vi "PicoScope4000aGetRapidBlockBulk.vi"(0 "error in":errorcluster, 3 "handle in":i16, 4 "Enabled array":i16[](array[numeric]), 5 "Rapid Block Acquisition Settings":T1) -> (6 "Channel A Buffer":i16[][](array[numeric]), 7 "Channel E Buffer":i16[][](array[numeric]), 8 "Channel B Buffer":i16[][](array[numeric]), 9 "Channel F Buffer":i16[][](array[numeric]), 10 "Channel C Buffer":i16[][](array[numeric]), 11 "Channel G Buffer":i16[][](array[numeric]), 12 "Channel D Buffer":i16[][](array[numeric]), 13 "Channel H Buffer":i16[][](array[numeric]), 14 "error out":errorcluster, 15 "handle out":i16, 16 "overflow":i16[](array[numeric]) format="%08b", 19 "Num samples":u32)   [LabVIEW 2009]
doc: "This VI gets a set of blocks captured using rapid block mode. It outputs two-dimensional arrays for each channel that contain data from all the requested captures."
uses:
  ps4000a.dll
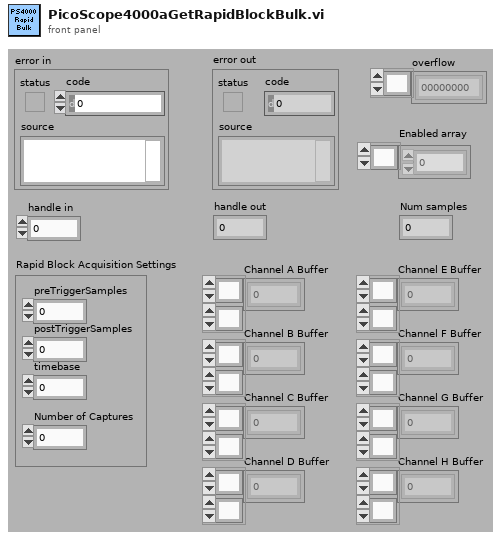
[diagram p1: front panel]
types:
  T1 = cluster{"preTriggerSamples":i32, "postTriggerSamples":i32, "timebase":u32, "Number of Captures":u32}
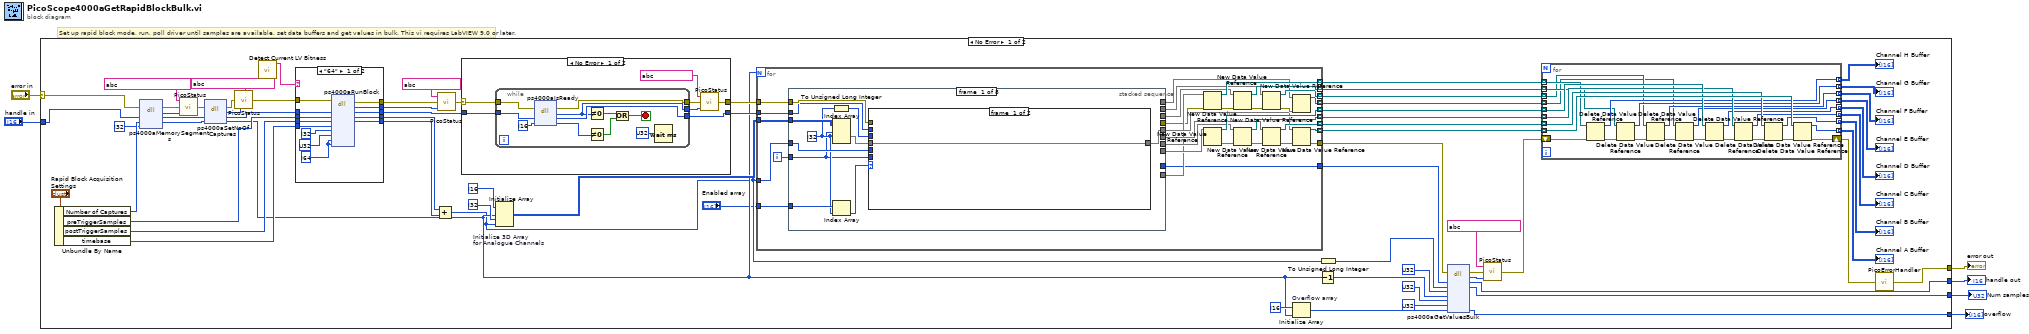
[diagram p0: block diagram]
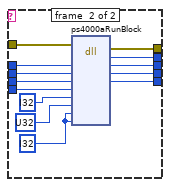
[diagram p2: hidden frame]
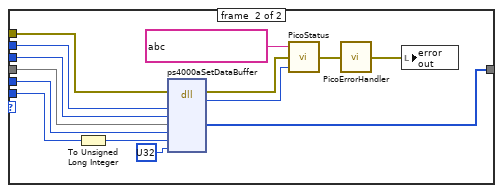
[diagram p3: hidden frame]
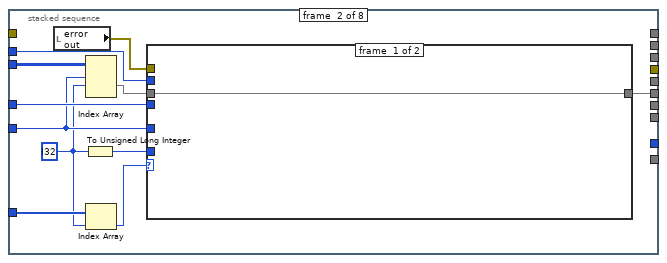
[diagram p4: hidden frame]
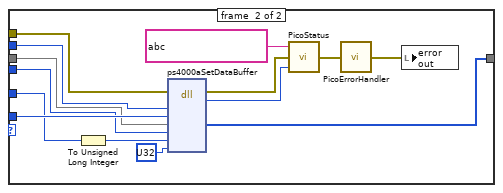
[diagram p5: hidden frame]
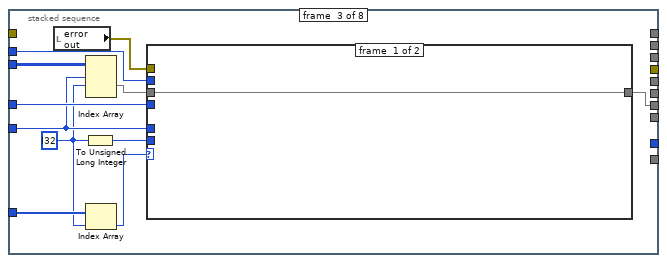
[diagram p6: hidden frame]
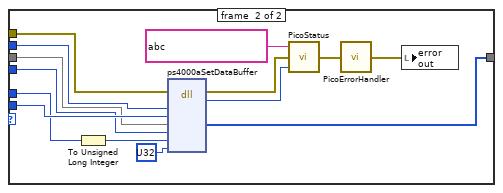
[diagram p7: hidden frame]
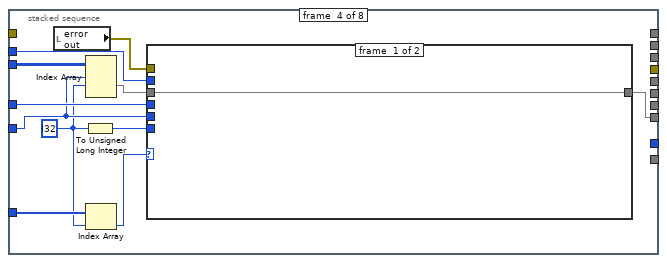
[diagram p8: hidden frame]
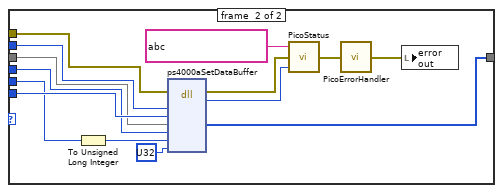
[diagram p9: hidden frame]
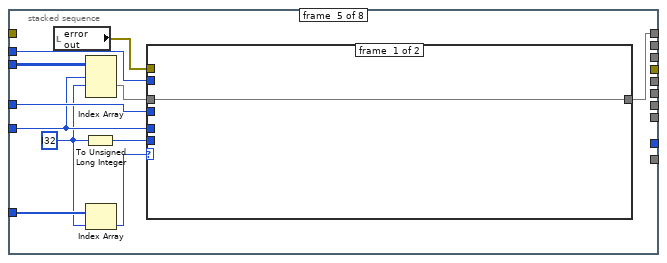
[diagram p10: hidden frame]
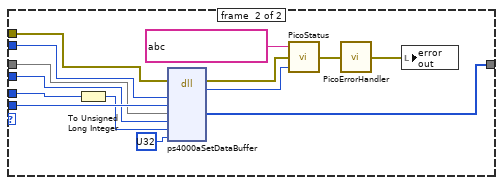
[diagram p11: hidden frame]
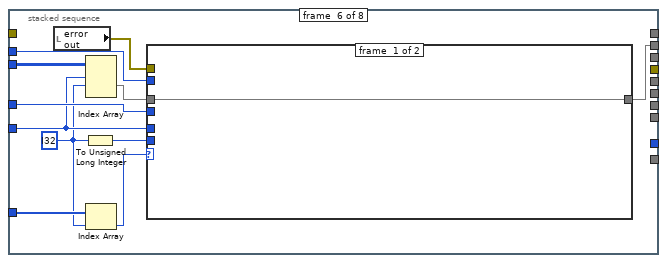
[diagram p12: hidden frame]
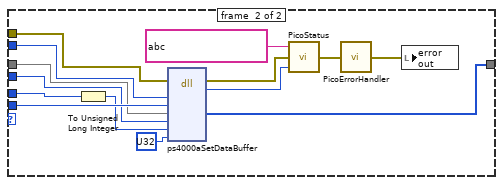
[diagram p13: hidden frame]
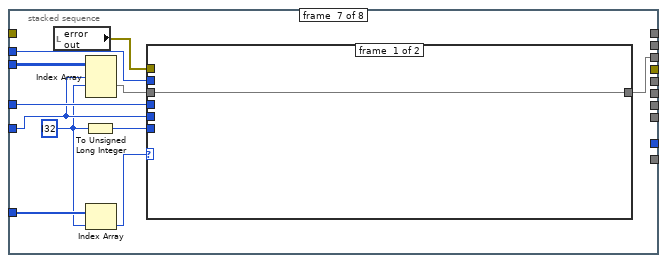
[diagram p14: hidden frame]
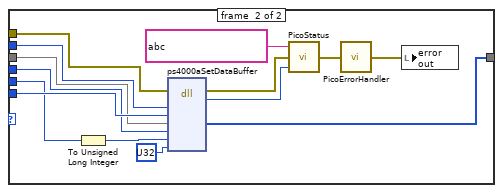
[diagram p15: hidden frame]
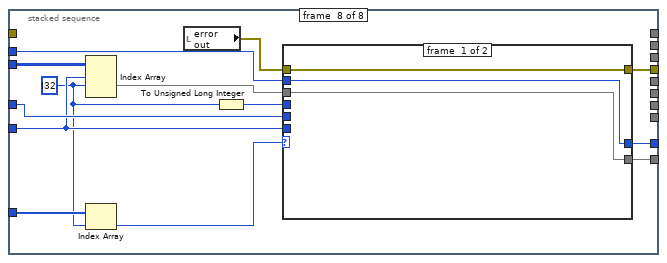
[diagram p16: hidden frame]
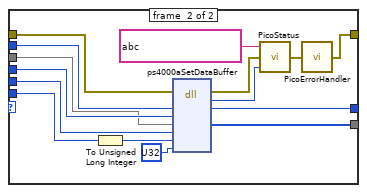
[diagram p17: hidden frame]
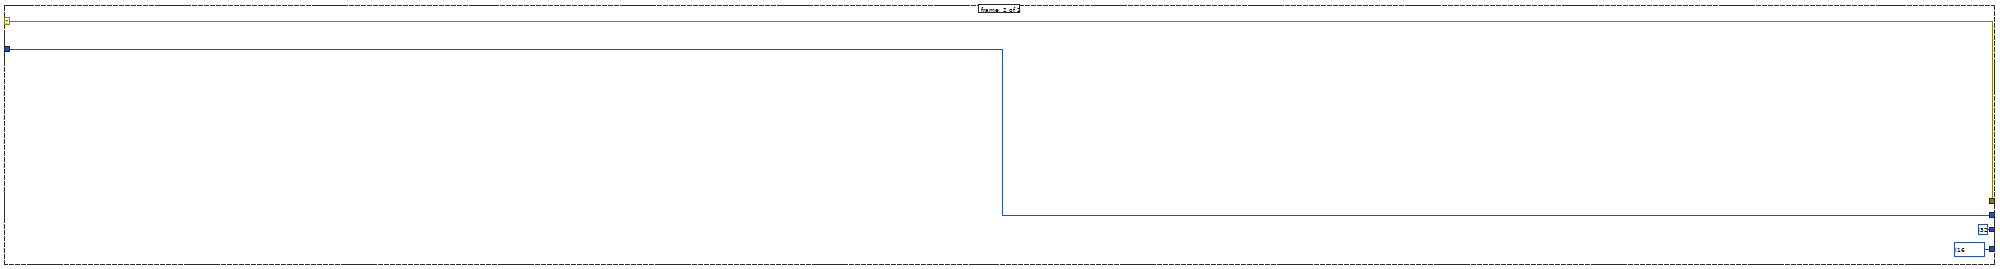
[diagram p19: hidden frame]
diagram:
  # "Set up rapid block mode, run, poll driver until samples are available, set data buffers and get values in bulk. This vi requires LabVIEW 9.0 or later."
  n1 = case shown="No Error" "error in" {
    selector: "error in" -> [w62 w394]
    tunnel: [w47 w394] -> w5
    tunnel: "handle in" -> [w61 w393]
    tunnel: [w37 w393] -> w3
    tunnel: [w19 i32 ?] -> w2
    tunnel: [w8 i16[] ? ("overflow")] -> w1
    frame #0 {
      n2 = Unbundle By Name("Rapid Block Acquisition Settings") -> ("Number of Captures"=w57:u32, "preTriggerSamples"=w68:i32, "postTriggerSamples"=w67:i32, "timebase"=w69:u32)
      n3 = dll-call lib="ps4000a.dll" fn="ps4000aMemorySegments" ("ps3000.dll:_ps3000_open_unit@0")(error in=w62, "handle"=w61, "nSegments"=w57, "nMaxSamples"=i32 ?) -> (error out=w59:errorcluster, "PICO_STATUS"=w60:u32, "handle"=w54:i16, "nSegments"=w55:u32)  [unwired: 3 in, 1 out]
      n4 = call "PicoStatus.vi"("PICO STATUS"=w60, "error in"=w59, "source"=string ?) -> ("error out"=w53:errorcluster)
      n5 = dll-call lib="ps4000a.dll" fn="ps4000aSetNoOfCaptures" ("ps3000.dll:_ps3000_open_unit@0")(error in=w53, "handle"=w54, "nCaptures"=w55) -> (error out=w51:errorcluster, "PICO_STATUS"=w52:u32, "handle"=w48:i16, "nCaptures"=w21:u32)  [unwired: 2 in, 1 out]
      n6 = call "PicoStatus.vi"("PICO STATUS"=w52, "error in"=w51, "source"=string ?) -> ("error out"=w49:errorcluster)
      n7 = call "Detect Current LV Bitness.vi"() -> ("bitness"=w7:string)  [unwired: 11 in]
      n8 = case shown="\"64\"" w7 {
        tunnel: [w88 w101] -> w75
        tunnel: [w87 w100] -> w73
        tunnel: [w86 w99] -> w72
        tunnel: w69 -> [w85 w98]
        tunnel: w68 -> [w84 w97]
        tunnel: w67 -> [w83 w96]
        tunnel: [w82 w95] -> w66
        tunnel: [w81 w94] -> w65
        tunnel: w49 -> [w80 w93]
        tunnel: w48 -> [w79 w92]
        frame #0 {
          w76 = i64 ? ("pParameter")
          n9 = dll-call lib="ps4000a.dll" fn="ps4000aRunBlock" ("ps3000.dll:_ps3000_open_unit@0")(error in=w80, "handle"=w79, "preTriggerSamples"=w84, "postTriggerSamples"=w83, "timebase"=w85, "timeindisposedMs"=i32 ? ("pParameter"), "segmentIndex"=u32 ? ("pParameter"), "lpReady"=w76, "pParameter"=w76) -> (error out=w81:errorcluster, "PICO_STATUS"=w82:u32, "handle"=w88:i16, "preTriggerSamples"=w87:i32, "postTriggerSamples"=w86:i32)  [unwired: 7 in, 1 out]
        }
        frame #1 {
          w89 = i32 ? ("pParameter")
          n10 = dll-call lib="ps4000a.dll" fn="ps4000aRunBlock" ("ps3000.dll:_ps3000_open_unit@0")(error in=w93, "handle"=w92, "preTriggerSamples"=w97, "postTriggerSamples"=w96, "timebase"=w98, "timeindisposedMs"=i32 ? ("pParameter"), "segmentIndex"=u32 ? ("pParameter"), "lpReady"=w89, "pParameter"=w89) -> (error out=w94:errorcluster, "PICO_STATUS"=w95:u32, "handle"=w101:i16, "preTriggerSamples"=w100:i32, "postTriggerSamples"=w99:i32)  [unwired: 7 in, 1 out]
        }
      }
      n11 = Add(x=w73, y=w72) -> (x+y=w20:i32)
      n12 = call "PicoStatus.vi"("PICO STATUS"=w66, "error in"=w65, "source"=string ?) -> ("error out"=w64:errorcluster)
      n13 = case shown="No Error" w64 {
        selector: w64 -> [w375 w389]
        tunnel: w75 -> [w377 w390]
        tunnel: [w376 w390] -> w74
        tunnel: [w374 w389] -> w71
        frame #0 {
          n14 = while {
            tunnel: [w388] -> w376
            tunnel: w377 -> [w387]
            tunnel: [w382] -> w372
            tunnel: w375 -> [w381]
            tunnel: [w380] -> w373
            stop <- w386 stop-if-true
            n15 = dll-call lib="ps4000a.dll" fn="ps4000aIsReady" ("ps3000.dll:_ps3000_open_unit@0")(error in=w381, "handle"=w387, "ready"=i16 ?) -> (error out=w380:errorcluster, "PICO_STATUS"=w382:u32, "handle"=w388:i16, "ready"=w383:i16)  [unwired: 2 in, 1 out]
            n16 = Not Equal To 0?(x=w382) -> (x != 0?=w384:bool)
            n17 = Not Equal To 0?(x=w383) -> (x != 0?=w385:bool)
            n18 = Or(x=w384, y=w385) -> (x .or. y?=w386:bool)
            n19 = Wait (ms)(milliseconds to wait=u32 ? ("ready")) -> ()  [unwired: 1 out]
          }
          n20 = call "PicoStatus.vi"("PICO STATUS"=w372, "error in"=w373, "source"=string ?) -> ("error out"=w374:errorcluster)
        }
        frame #1 {
        }
      }
      n21 = Initialize Array "Initialize 3D Array\nfor Analogue Channels"(i16 ? ("element"), w21, i32 ? ("dimension size"), w20) -> (w22:i16[][][])
      n22 = for {
        N: w21 -> [_]
        tunnel: w74 -> [w137]
        tunnel: w71 -> [w141]
        tunnel: [w150] -> w36
        tunnel: [w154] -> w35 mode=indexing
        tunnel: [w153] -> w34 mode=indexing
        tunnel: [w152] -> w33 mode=indexing
        tunnel: [w151] -> w32 mode=indexing
        tunnel: [w127] -> w28
        tunnel: w22 -> [w139]
        tunnel: w20 -> [w138]
        tunnel: [w146] -> w13 mode=indexing
        tunnel: [w145] -> w12 mode=indexing
        tunnel: [w144] -> w11 mode=indexing
        tunnel: [w143] -> w10 mode=indexing
        tunnel: "Enabled array" -> [w142]
        i -> [w140]
        n23 = stacked-sequence {
          tunnel: [w166 _ _ _ _ _ _ _] -> w136
          tunnel: w142 -> [w168 w194 w220 w246 w272 w298 w324 w352]
          tunnel: w141 -> [w164 _ _ _ _ _ _ _]
          tunnel: w140 -> [w158 w186 w212 w238 w264 w290 w316 w344]
          tunnel: w139 -> [w163 w191 w217 w243 w269 w295 w321 w349]
          tunnel: w138 -> [w161 w189 w215 w241 w267 w293 w319 w347]
          tunnel: w137 -> [w160 w188 w214 w240 w266 w292 w318 w346]
          tunnel: [_ w184 _ _ _ _ _ _] -> w135
          tunnel: [_ _ w210 _ _ _ _ _] -> w134
          tunnel: [_ _ _ w236 _ _ _ _] -> w133
          tunnel: [_ _ _ _ w262 _ _ _] -> w132
          tunnel: [_ _ _ _ _ w288 _ _] -> w131
          tunnel: [_ _ _ _ _ _ w314 _] -> w130
          tunnel: [_ _ _ _ _ _ _ w342] -> w129
          tunnel: [_ _ _ _ _ _ _ w341] -> w128
          tunnel: [_ _ _ _ _ _ _ w340] -> w127
          frame #0 {
            w159 = i32 ? ("index")
            n24 = To Unsigned Long Integer(number=w159) -> (unsigned 32bit integer=w165:u32)
            n25 = Index Array(array=w163, index (dim 0)=w158, index (dim 1)=w159) -> (element=w162:i16[])  [unwired: 1 in]
            n26 = Index Array(array=w168, index=w159) -> (element=w167:i16)
            n27 = case shown="1" w167 {
              tunnel: w164 -> [_ w180]
              tunnel: [w169 w179] -> w166
              tunnel: w165 -> [_ w176]
              tunnel: w162 -> [w169 w174]
              tunnel: w161 -> [_ w173]
              tunnel: w158 -> [_ w172]
              tunnel: w160 -> [_ w170]
              frame #0 {
              }
              frame #1 {
                n28 = To Unsigned Long Integer(number=w172) -> (unsigned 32bit integer=w171:u32)
                n29 = dll-call lib="ps4000a.dll" fn="ps4000aSetDataBuffer" ("ps3000.dll:_ps3000_open_unit@0")(error in=w180, "handle"=w170, "channel"=w176, "buffer"=w174, "bufferLth"=w173, "segmentIndex"=w171, "mode"=u32 ?) -> (error out=w183:errorcluster, "PICO_STATUS"=w182:u32, "buffer"=w179:i16[])  [unwired: 7 in, 1 out]
                n30 = call "PicoStatus.vi"("PICO STATUS"=w182, "error in"=w183, "source"=string ?) -> ("error out"=w178:errorcluster)
                n31 = call "PicoErrorHandler.vi"("error in"=w178) -> ("error out"=w175:errorcluster)
                n32 = local write "error out"(w175) -> ()
              }
            }
          }
          frame #1 {
            w185 = i32 ? ("index")
            n33 = local read "error out"() -> (w187:errorcluster)
            n34 = To Unsigned Long Integer(number=w185) -> (unsigned 32bit integer=w192:u32)
            n35 = Index Array(array=w191, index (dim 0)=w186, index (dim 1)=w185) -> (element=w190:i16[])  [unwired: 1 in]
            n36 = Index Array(array=w194, index=w185) -> (element=w193:i16)
            n37 = case shown="1" w193 {
              tunnel: w187 -> [_ w206]
              tunnel: [w195 w205] -> w184
              tunnel: w192 -> [_ w202]
              tunnel: w190 -> [w195 w200]
              tunnel: w189 -> [_ w199]
              tunnel: w186 -> [_ w198]
              tunnel: w188 -> [_ w196]
              frame #0 {
              }
              frame #1 {
                n38 = To Unsigned Long Integer(number=w198) -> (unsigned 32bit integer=w197:u32)
                n39 = dll-call lib="ps4000a.dll" fn="ps4000aSetDataBuffer" ("ps3000.dll:_ps3000_open_unit@0")(error in=w206, "handle"=w196, "channel"=w202, "buffer"=w200, "bufferLth"=w199, "segmentIndex"=w197, "mode"=u32 ?) -> (error out=w209:errorcluster, "PICO_STATUS"=w208:u32, "buffer"=w205:i16[])  [unwired: 7 in, 1 out]
                n40 = call "PicoStatus.vi"("PICO STATUS"=w208, "error in"=w209, "source"=string ?) -> ("error out"=w204:errorcluster)
                n41 = call "PicoErrorHandler.vi"("error in"=w204) -> ("error out"=w201:errorcluster)
                n42 = local write "error out"(w201) -> ()
              }
            }
          }
          frame #2 {
            w211 = i32 ? ("index")
            n43 = local read "error out"() -> (w213:errorcluster)
            n44 = To Unsigned Long Integer(number=w211) -> (unsigned 32bit integer=w218:u32)
            n45 = Index Array(array=w217, index (dim 0)=w212, index (dim 1)=w211) -> (element=w216:i16[])  [unwired: 1 in]
            n46 = Index Array(array=w220, index=w211) -> (element=w219:i16)
            n47 = case shown="1" w219 {
              tunnel: w213 -> [_ w232]
              tunnel: [w221 w231] -> w210
              tunnel: w218 -> [_ w228]
              tunnel: w216 -> [w221 w226]
              tunnel: w215 -> [_ w225]
              tunnel: w212 -> [_ w224]
              tunnel: w214 -> [_ w222]
              frame #0 {
              }
              frame #1 {
                n48 = To Unsigned Long Integer(number=w224) -> (unsigned 32bit integer=w223:u32)
                n49 = dll-call lib="ps4000a.dll" fn="ps4000aSetDataBuffer" ("ps3000.dll:_ps3000_open_unit@0")(error in=w232, "handle"=w222, "channel"=w228, "buffer"=w226, "bufferLth"=w225, "segmentIndex"=w223, "mode"=u32 ?) -> (error out=w235:errorcluster, "PICO_STATUS"=w234:u32, "buffer"=w231:i16[])  [unwired: 7 in, 1 out]
                n50 = call "PicoStatus.vi"("PICO STATUS"=w234, "error in"=w235, "source"=string ?) -> ("error out"=w230:errorcluster)
                n51 = call "PicoErrorHandler.vi"("error in"=w230) -> ("error out"=w227:errorcluster)
                n52 = local write "error out"(w227) -> ()
              }
            }
          }
          frame #3 {
            w237 = i32 ? ("index")
            n53 = local read "error out"() -> (w239:errorcluster)
            n54 = To Unsigned Long Integer(number=w237) -> (unsigned 32bit integer=w244:u32)
            n55 = Index Array(array=w243, index (dim 0)=w238, index (dim 1)=w237) -> (element=w242:i16[])  [unwired: 1 in]
            n56 = Index Array(array=w246, index=w237) -> (element=w245:i16)
            n57 = case shown="1" w245 {
              tunnel: w239 -> [_ w258]
              tunnel: [w247 w257] -> w236
              tunnel: w244 -> [_ w254]
              tunnel: w242 -> [w247 w252]
              tunnel: w241 -> [_ w251]
              tunnel: w238 -> [_ w250]
              tunnel: w240 -> [_ w248]
              frame #0 {
              }
              frame #1 {
                n58 = To Unsigned Long Integer(number=w250) -> (unsigned 32bit integer=w249:u32)
                n59 = dll-call lib="ps4000a.dll" fn="ps4000aSetDataBuffer" ("ps3000.dll:_ps3000_open_unit@0")(error in=w258, "handle"=w248, "channel"=w254, "buffer"=w252, "bufferLth"=w251, "segmentIndex"=w249, "mode"=u32 ?) -> (error out=w261:errorcluster, "PICO_STATUS"=w260:u32, "buffer"=w257:i16[])  [unwired: 7 in, 1 out]
                n60 = call "PicoStatus.vi"("PICO STATUS"=w260, "error in"=w261, "source"=string ?) -> ("error out"=w256:errorcluster)
                n61 = call "PicoErrorHandler.vi"("error in"=w256) -> ("error out"=w253:errorcluster)
                n62 = local write "error out"(w253) -> ()
              }
            }
          }
          frame #4 {
            w263 = i32 ? ("index")
            n63 = local read "error out"() -> (w265:errorcluster)
            n64 = To Unsigned Long Integer(number=w263) -> (unsigned 32bit integer=w270:u32)
            n65 = Index Array(array=w269, index (dim 0)=w264, index (dim 1)=w263) -> (element=w268:i16[])  [unwired: 1 in]
            n66 = Index Array(array=w272, index=w263) -> (element=w271:i16)
            n67 = case shown="1" w271 {
              tunnel: w265 -> [_ w284]
              tunnel: [w273 w283] -> w262
              tunnel: w270 -> [_ w280]
              tunnel: w268 -> [w273 w278]
              tunnel: w267 -> [_ w277]
              tunnel: w264 -> [_ w276]
              tunnel: w266 -> [_ w274]
              frame #0 {
              }
              frame #1 {
                n68 = To Unsigned Long Integer(number=w276) -> (unsigned 32bit integer=w275:u32)
                n69 = dll-call lib="ps4000a.dll" fn="ps4000aSetDataBuffer" ("ps3000.dll:_ps3000_open_unit@0")(error in=w284, "handle"=w274, "channel"=w280, "buffer"=w278, "bufferLth"=w277, "segmentIndex"=w275, "mode"=u32 ?) -> (error out=w287:errorcluster, "PICO_STATUS"=w286:u32, "buffer"=w283:i16[])  [unwired: 7 in, 1 out]
                n70 = call "PicoStatus.vi"("PICO STATUS"=w286, "error in"=w287, "source"=string ?) -> ("error out"=w282:errorcluster)
                n71 = call "PicoErrorHandler.vi"("error in"=w282) -> ("error out"=w279:errorcluster)
                n72 = local write "error out"(w279) -> ()
              }
            }
          }
          frame #5 {
            w289 = i32 ? ("index")
            n73 = local read "error out"() -> (w291:errorcluster)
            n74 = To Unsigned Long Integer(number=w289) -> (unsigned 32bit integer=w296:u32)
            n75 = Index Array(array=w295, index (dim 0)=w290, index (dim 1)=w289) -> (element=w294:i16[])  [unwired: 1 in]
            n76 = Index Array(array=w298, index=w289) -> (element=w297:i16)
            n77 = case shown="1" w297 {
              tunnel: w291 -> [_ w310]
              tunnel: [w299 w309] -> w288
              tunnel: w296 -> [_ w306]
              tunnel: w294 -> [w299 w304]
              tunnel: w293 -> [_ w303]
              tunnel: w290 -> [_ w302]
              tunnel: w292 -> [_ w300]
              frame #0 {
              }
              frame #1 {
                n78 = To Unsigned Long Integer(number=w302) -> (unsigned 32bit integer=w301:u32)
                n79 = dll-call lib="ps4000a.dll" fn="ps4000aSetDataBuffer" ("ps3000.dll:_ps3000_open_unit@0")(error in=w310, "handle"=w300, "channel"=w306, "buffer"=w304, "bufferLth"=w303, "segmentIndex"=w301, "mode"=u32 ?) -> (error out=w313:errorcluster, "PICO_STATUS"=w312:u32, "buffer"=w309:i16[])  [unwired: 7 in, 1 out]
                n80 = call "PicoStatus.vi"("PICO STATUS"=w312, "error in"=w313, "source"=string ?) -> ("error out"=w308:errorcluster)
                n81 = call "PicoErrorHandler.vi"("error in"=w308) -> ("error out"=w305:errorcluster)
                n82 = local write "error out"(w305) -> ()
              }
            }
          }
          frame #6 {
            w315 = i32 ? ("index")
            n83 = local read "error out"() -> (w317:errorcluster)
            n84 = To Unsigned Long Integer(number=w315) -> (unsigned 32bit integer=w322:u32)
            n85 = Index Array(array=w321, index (dim 0)=w316, index (dim 1)=w315) -> (element=w320:i16[])  [unwired: 1 in]
            n86 = Index Array(array=w324, index=w315) -> (element=w323:i16)
            n87 = case shown="1" w323 {
              tunnel: w317 -> [_ w336]
              tunnel: [w325 w335] -> w314
              tunnel: w322 -> [_ w332]
              tunnel: w320 -> [w325 w330]
              tunnel: w319 -> [_ w329]
              tunnel: w316 -> [_ w328]
              tunnel: w318 -> [_ w326]
              frame #0 {
              }
              frame #1 {
                n88 = To Unsigned Long Integer(number=w328) -> (unsigned 32bit integer=w327:u32)
                n89 = dll-call lib="ps4000a.dll" fn="ps4000aSetDataBuffer" ("ps3000.dll:_ps3000_open_unit@0")(error in=w336, "handle"=w326, "channel"=w332, "buffer"=w330, "bufferLth"=w329, "segmentIndex"=w327, "mode"=u32 ?) -> (error out=w339:errorcluster, "PICO_STATUS"=w338:u32, "buffer"=w335:i16[])  [unwired: 7 in, 1 out]
                n90 = call "PicoStatus.vi"("PICO STATUS"=w338, "error in"=w339, "source"=string ?) -> ("error out"=w334:errorcluster)
                n91 = call "PicoErrorHandler.vi"("error in"=w334) -> ("error out"=w331:errorcluster)
                n92 = local write "error out"(w331) -> ()
              }
            }
          }
          frame #7 {
            w343 = i32 ? ("index")
            n93 = Index Array(array=w349, index (dim 0)=w344, index (dim 1)=w343) -> (element=w348:i16[])  [unwired: 1 in]
            n94 = Index Array(array=w352, index=w343) -> (element=w351:i16)
            n95 = local read "error out"() -> (w345:errorcluster)
            n96 = To Unsigned Long Integer(number=w343) -> (unsigned 32bit integer=w350:u32)
            n97 = case shown="1" w351 {
              tunnel: w345 -> [w354 w367]
              tunnel: [w355 w366] -> w342
              tunnel: w350 -> [_ w363]
              tunnel: w348 -> [w355 w362]
              tunnel: w347 -> [_ w361]
              tunnel: w344 -> [_ w360]
              tunnel: w346 -> [w353 w358]
              tunnel: [w354 w357] -> w341
              tunnel: [w353 w356] -> w340
              frame #0 {
              }
              frame #1 {
                n98 = To Unsigned Long Integer(number=w360) -> (unsigned 32bit integer=w359:u32)
                n99 = dll-call lib="ps4000a.dll" fn="ps4000aSetDataBuffer" ("ps3000.dll:_ps3000_open_unit@0")(error in=w367, "handle"=w358, "channel"=w363, "buffer"=w362, "bufferLth"=w361, "segmentIndex"=w359, "mode"=u32 ?) -> (error out=w370:errorcluster, "PICO_STATUS"=w369:u32, "handle"=w356:i16, "buffer"=w366:i16[])  [unwired: 6 in, 1 out]
                n100 = call "PicoStatus.vi"("PICO STATUS"=w369, "error in"=w370, "source"=string ?) -> ("error out"=w365:errorcluster)
                n101 = call "PicoErrorHandler.vi"("error in"=w365) -> ("error out"=w357:errorcluster)
              }
            }
          }
        }
        n102 = New Data Value Reference(data value=w129, error in=w128) -> (data value reference=w146:refnum<data-value>, error out=w149:errorcluster)
        n103 = New Data Value Reference(data value=w133) -> (data value reference=w154:refnum<data-value>, error out=w157:errorcluster)  [unwired: 1 in]
        n104 = New Data Value Reference(data value=w130, error in=w149) -> (data value reference=w145:refnum<data-value>, error out=w148:errorcluster)
        n105 = New Data Value Reference(data value=w134, error in=w157) -> (data value reference=w153:refnum<data-value>, error out=w156:errorcluster)
        n106 = New Data Value Reference(data value=w131, error in=w148) -> (data value reference=w144:refnum<data-value>, error out=w147:errorcluster)
        n107 = New Data Value Reference(data value=w135, error in=w156) -> (data value reference=w152:refnum<data-value>, error out=w155:errorcluster)
        n108 = New Data Value Reference(data value=w132, error in=w147) -> (data value reference=w143:refnum<data-value>)  [unwired: 1 out]
        n109 = New Data Value Reference(data value=w136, error in=w155) -> (data value reference=w151:refnum<data-value>, error out=w150:errorcluster)
      }
      n110 = Initialize Array "Overflow array"(i16 ? ("element"), w21) -> (w25:i16[])
      n111 = To Unsigned Long Integer(number=w20) -> (unsigned 32bit integer=w18:u32)
      n112 = Decrement(x=w21) -> (x-1=w27:u32)
      n113 = dll-call lib="ps4000a.dll" fn="ps4000aGetValuesBulk" ("ps3000.dll:_ps3000_open_unit@0")(error in=w36, "handle"=w28, "noOfSamples"=w18, "fromSegmentIndex"=u32 ?, "toSegmentIndex"=w27, "downSampleRatio"=u32 ?, "downSampleRatioMode"=u32 ?, "overflow"=w25) -> (error out=w40:errorcluster, "PICO_STATUS"=w39:u32, "handle"=w37:i16, "noOfSamples"=w19:u32, "overflow"=w8:i16[])  [unwired: 6 in, 1 out]
      n114 = call "PicoStatus.vi"("PICO STATUS"=w39, "error in"=w40, "source"=string ?) -> ("error out"=w38:errorcluster)
      n115 = for {
        tunnel: w32 -> [w126] mode=indexing
        tunnel: [w125] -> w41 mode=indexing
        shift-right: [w115] -> w45
        shift-left: w38 -> [w114]
        tunnel: w33 -> [w124] mode=indexing
        tunnel: w35 -> [w123] mode=indexing
        tunnel: w34 -> [w122] mode=indexing
        tunnel: [w118] -> w44 mode=indexing
        tunnel: [w117] -> w43 mode=indexing
        tunnel: [w116] -> w42 mode=indexing
        tunnel: [w109] -> w17 mode=indexing
        tunnel: [w108] -> w16 mode=indexing
        tunnel: [w107] -> w15 mode=indexing
        tunnel: [w106] -> w14 mode=indexing
        tunnel: w13 -> [w105] mode=indexing
        tunnel: w12 -> [w104] mode=indexing
        tunnel: w11 -> [w103] mode=indexing
        tunnel: w10 -> [w102] mode=indexing
        n116 = Delete Data Value Reference(data value reference=w105, error in=w114) -> (data value=w109:i16[], error out=w113:errorcluster)
        n117 = Delete Data Value Reference(data value reference=w104, error in=w113) -> (data value=w108:i16[], error out=w112:errorcluster)
        n118 = Delete Data Value Reference(data value reference=w103, error in=w112) -> (data value=w107:i16[], error out=w111:errorcluster)
        n119 = Delete Data Value Reference(data value reference=w102, error in=w111) -> (data value=w106:i16[], error out=w110:errorcluster)
        n120 = Delete Data Value Reference(data value reference=w123, error in=w110) -> (data value=w118:i16[], error out=w121:errorcluster)
        n121 = Delete Data Value Reference(data value reference=w122, error in=w121) -> (data value=w117:i16[], error out=w120:errorcluster)
        n122 = Delete Data Value Reference(data value reference=w124, error in=w120) -> (data value=w116:i16[], error out=w119:errorcluster)
        n123 = Delete Data Value Reference(data value reference=w126, error in=w119) -> (data value=w125:i16[], error out=w115:errorcluster)
      }
      "Channel D Buffer" <- w44
      "Channel C Buffer" <- w43
      "Channel B Buffer" <- w42
      "Channel A Buffer" <- w41
      "Channel H Buffer" <- w17
      "Channel G Buffer" <- w16
      "Channel F Buffer" <- w15
      "Channel E Buffer" <- w14
      n124 = call "PicoErrorHandler.vi"("error in"=w45) -> ("error out"=w47:errorcluster)
    }
    frame #1 {
    }
  }
  "error out" <- w5
  "handle out" <- w3
  "Num samples" <- w2
  "overflow" <- w1
